vi "aggregator - iii - complex.vi"(5 "requested averaging interval":i32=10, 6 "first time":bool, 7 "requested size":i32=20, 11 "number":cdb) -> (0 "interpolated average":cdb, 1 "mean array":cdb[](array[numeric]), 2 "interp array":cdb[](array[numeric]), 3 "Array":cdb[](array[numeric]), 4 "slope":cdb)   [LabVIEW 2012]
panel:
  out "actual number of elements":i32
  out "mean":cdb
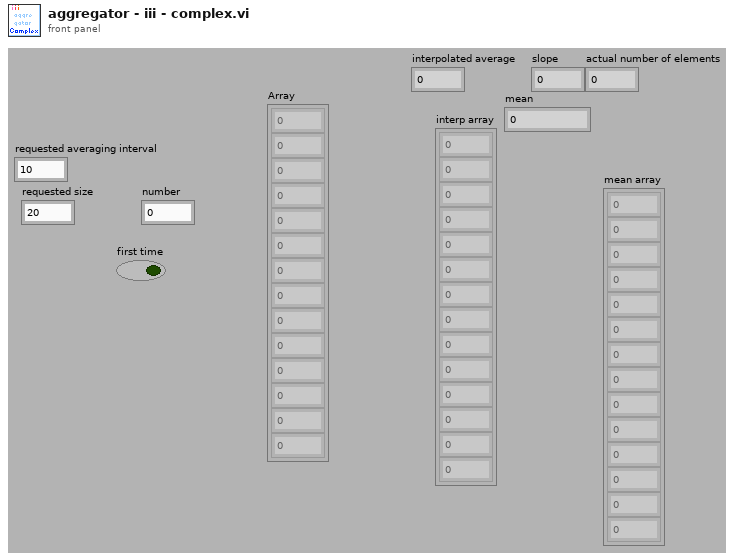
[diagram p1: front panel]
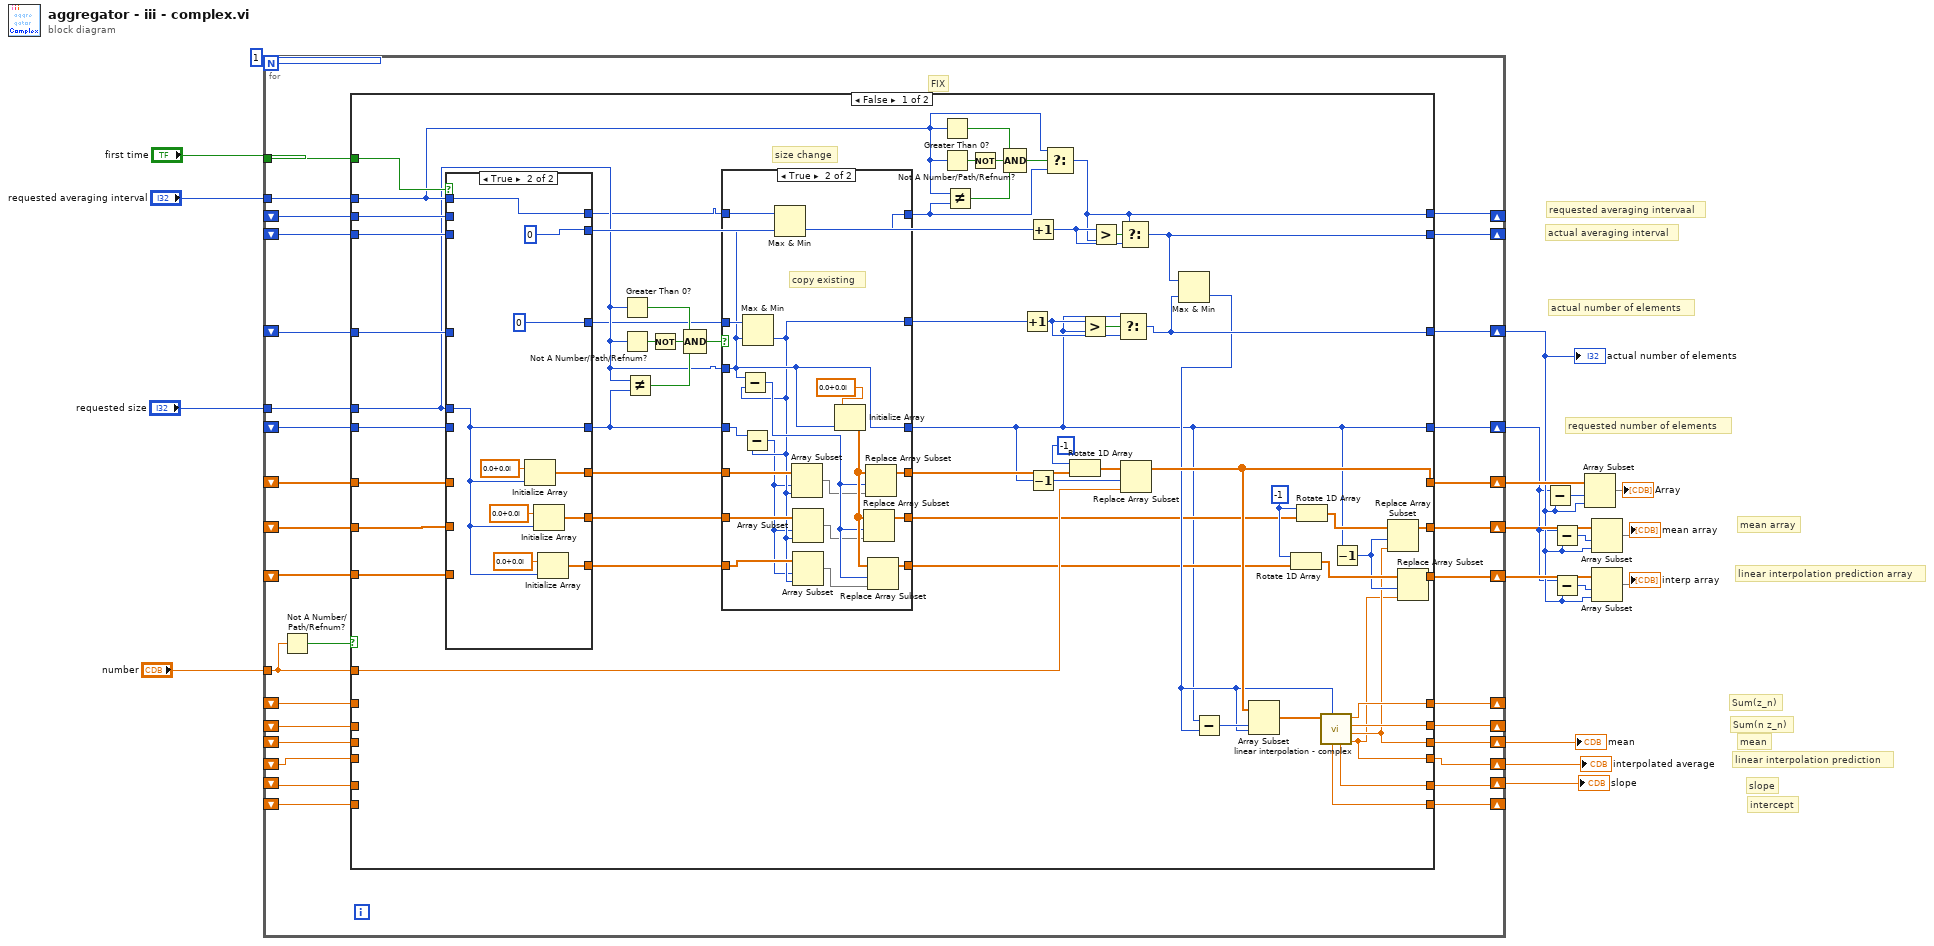
[diagram p0: block diagram]
diagram:
  # "actual averaging interval"
  # "requested averaging intervaal"
  # "linear interpolation prediction"
  # "mean"
  # "intercept"
  # "slope"
  # "linear interpolation prediction array"
  # "mean array"
  # "Sum(n z_n)"
  # "Sum(z_n)"
  # "requested number of elements"
  # "actual number of elements"
  n1 = for {
    N: 1 -> [_]
    tunnel: "first time" -> [w40]
    shift-right: [w29] -> w5
    shift-left: _ -> [w50]
    tunnel: "requested size" -> [w33]
    tunnel: "number" -> [w27]
    shift-right: [w41] -> w15
    shift-left: _ -> [w49]
    shift-right: [w32] -> w4
    shift-left: _ -> [w48]
    shift-right: [w45] -> w9
    shift-left: _ -> [w47]
    shift-right: [w44] -> w6
    shift-left: _ -> [w46]
    shift-right: [w39] -> _
    shift-left: _ -> [w25]
    shift-right: [w38] -> _
    shift-left: _ -> [w24]
    shift-right: [w35] -> w2
    shift-left: _ -> [w21]
    shift-right: [w34] -> _
    shift-left: _ -> [w20]
    shift-right: [w37] -> w1
    shift-left: _ -> [w23]
    shift-right: [w36] -> w3
    shift-left: _ -> [w22]
    shift-right: [w28] -> _
    shift-left: _ -> [w43]
    shift-right: [w30] -> _
    shift-left: _ -> [w42]
    tunnel: "requested averaging interval" -> [w31]
    # "FIX"
    n2 = Not A Number/Path/Refnum?(number/path/refnum=w27) -> (NaN/Path/Refnum?=w26:bool)
    n3 = case shown="False" w26 {
      tunnel: w50 -> [w110 w163]
      tunnel: w49 -> [w107 w161]
      tunnel: w27 -> [w105 _]
      tunnel: w48 -> [w102 w162]
      tunnel: w47 -> [w101 w160]
      tunnel: w46 -> [w100 w153]
      tunnel: [w95 w160] -> w45
      tunnel: [w94 w153] -> w44
      tunnel: w43 -> [w90 w164]
      tunnel: w42 -> [w89 w165]
      tunnel: [w88 w161] -> w41
      tunnel: w40 -> [w86 _]
      tunnel: [w84 w159] -> w39
      tunnel: [w83 w158] -> w38
      tunnel: [w82 w157] -> w37
      tunnel: [w81 w156] -> w36
      tunnel: [w80 w155] -> w35
      tunnel: [w79 w154] -> w34
      tunnel: w33 -> [w56 _]
      tunnel: [w57 w162] -> w32
      tunnel: w31 -> [w69 _]
      tunnel: [w68 w165] -> w30
      tunnel: [w67 w163] -> w29
      tunnel: [w66 w164] -> w28
      tunnel: w25 -> [_ w159]
      tunnel: w24 -> [_ w158]
      tunnel: w23 -> [_ w157]
      tunnel: w22 -> [_ w156]
      tunnel: w21 -> [_ w155]
      tunnel: w20 -> [_ w154]
      frame False {
        w97 = -1 ("n")
        # "size change"
        n4 = case shown="True" w86 {
          tunnel: w110 -> [w141 _]
          tunnel: [w141 0] -> w54
          tunnel: w107 -> [w138 _]
          tunnel: w56 -> [_ w143]
          tunnel: w102 -> [w139 _]
          tunnel: w101 -> [w137 _]
          tunnel: w100 -> [w136 _]
          tunnel: [w138 w146] -> w59
          tunnel: [w137 w145] -> w60
          tunnel: [w136 w144] -> w61
          tunnel: [w142 0] -> w92
          tunnel: w90 -> [w142 _]
          tunnel: w69 -> [_ w147]
          tunnel: w89 -> [w140 _]
          tunnel: [w140 w147] -> w53
          tunnel: [w139 w143] -> w58
          frame False {
          }
          frame True {
            n5 = Initialize Array(cdb 0.0+0.0i, w143) -> (w146:cdb[])
            n6 = Initialize Array(cdb 0.0+0.0i, w143) -> (w145:cdb[])
            n7 = Initialize Array(cdb 0.0+0.0i, w143) -> (w144:cdb[])
          }
        }
        n8 = Greater Than 0?(x=w56) -> (x > 0?=w77:bool)
        n9 = Not A Number/Path/Refnum?(number/path/refnum=w56) -> (NaN/Path/Refnum?=w78:bool)
        n10 = Not Equal?(x=w56, y=w58) -> (x != y?=w75:bool)
        n11 = Not(x=w78) -> (.not. x?=w76:bool)
        n12 = Compound Arithmetic op=AND(w77, w76, w75) -> (w55:bool)
        n13 = case shown="True" w55 {
          tunnel: [w116 w118] -> w51
          tunnel: w54 -> [w116 w134]
          tunnel: [w115 w126] -> w57
          tunnel: w58 -> [w115 w119]
          tunnel: [w114 w133] -> w64
          tunnel: w59 -> [w114 w125]
          tunnel: w56 -> [_ w126]
          tunnel: w61 -> [w112 w123]
          tunnel: w60 -> [w113 w121]
          tunnel: [w113 w132] -> w63
          tunnel: [w112 w131] -> w62
          tunnel: w53 -> [w111 w128]
          tunnel: [w111 w127] -> w52
          frame False {
          }
          frame True {
            # "copy existing"
            n14 = Max & Min(x=w134, y=w126) -> (min(x,y)=w118:i32)  [unwired: 1 out]
            n15 = Subtract(x=w126, y=w118) -> (x-y=w129:i32)
            n16 = Subtract(x=w119, y=w118) -> (x-y=w117:i32)
            n17 = Max & Min(x=w128, y=w126) -> (min(x,y)=w127:i32)  [unwired: 1 out]
            n18 = Array Subset(array=w125, index=w117, length=w118) -> (w124:cdb[])
            n19 = Array Subset(array=w121, index=w117, length=w118) -> (w120:cdb[])
            n20 = Array Subset(array=w123, index=w117, length=w118) -> (w122:cdb[])
            n21 = Initialize Array(cdb 0.0+0.0i, w126) -> (w130:cdb[])
            n22 = Replace Array Subset(array=w130, new element=w120, index=w129) -> (w132:cdb[])
            n23 = Replace Array Subset(array=w130, new element=w124, index=w129) -> (w133:cdb[])
            n24 = Replace Array Subset(array=w130, new element=w122, index=w129) -> (w131:cdb[])
          }
        }
        n25 = Greater Than 0?(x=w69) -> (x > 0?=w73:bool)
        n26 = Not A Number/Path/Refnum?(number/path/refnum=w69) -> (NaN/Path/Refnum?=w74:bool)
        n27 = Not Equal?(x=w69, y=w52) -> (x != y?=w71:bool)
        n28 = Not(x=w74) -> (.not. x?=w72:bool)
        n29 = Compound Arithmetic op=AND(w73, w72, w71) -> (w70:bool)
        n30 = Increment(x=w51) -> (x+1=w108:i32)
        n31 = Increment(x=w92) -> (x+1=w91:i32)
        n32 = Decrement(x=w57) -> (x-1=w104:i32)
        n33 = Select(t=w69, s=w70, f=w52) -> (s? t:f=w68:i32)
        n34 = Rotate 1D Array(1:w64, 2:-1 ("n")) -> (0:w103:cdb[])
        n35 = Greater?(x=w108, y=w57) -> (0:w109:bool)
        n36 = Greater?(x=w91, y=w68) -> (0:w93:bool)
        n37 = Select(t=w57, s=w109, f=w108) -> (s? t:f=w67:i32)
        n38 = Select(t=w68, s=w93, f=w91) -> (s? t:f=w66:i32)
        n39 = Replace Array Subset(array=w103, new element=w105, index=w104) -> (w88:cdb[])
        n40 = Max & Min(x=w66, y=w67) -> (min(x,y)=w65:i32)  [unwired: 1 out]
        n41 = Subtract(x=w57, y=w65) -> (x-y=w87:i32)
        n42 = Array Subset(array=w88, index=w87, length=w65) -> (w85:cdb[])
        n43 = Rotate 1D Array(1:w62, 2:w97) -> (0:w98:cdb[])
        n44 = Rotate 1D Array(1:w63, 2:w97) -> (0:w99:cdb[])
        n45 = call "linear interpolation - complex.vi"("n"=w65, "Array"=w85) -> ("interpolated average"=w81:cdb, "mean"=w82:cdb, "sum n z_n"=w83:cdb, "sum z_n"=w84:cdb, "slope"=w80:cdb, "intercept"=w79:cdb)  [unwired: 3 in, 1 out]
        n46 = Decrement(x=w57) -> (x-1=w96:i32)
        n47 = Replace Array Subset(array=w99, new element=w82, index=w96) -> (w95:cdb[])
        n48 = Replace Array Subset(array=w98, new element=w81, index=w96) -> (w94:cdb[])
      }
      frame True {
      }
    }
  }
  "interpolated average" <- w3
  "slope" <- w2
  "mean" <- w1
  "actual number of elements" <- w5
  n49 = Subtract(x=w4, y=w5) -> (x-y=w13:i32)
  n50 = Subtract(x=w4, y=w5) -> (x-y=w10:i32)
  n51 = Subtract(x=w4, y=w5) -> (x-y=w7:i32)
  n52 = Array Subset(array=w15, index=w13, length=w5) -> (→"Array":cdb[])
  n53 = Array Subset(array=w9, index=w10, length=w5) -> (→"mean array":cdb[])
  n54 = Array Subset(array=w6, index=w7, length=w5) -> (→"interp array":cdb[])
